vi "Pointcloud Paint.vi"(8 "error in (no error)":errorcluster, 11 "Pointcloud in":refnum<class "Pointcloud.lvclass">) -> (0 "error out":errorcluster, 2 "Pointcloud":refnum<vi>, 3 "Pointcloud out":refnum<class "Pointcloud.lvclass">)   [LabVIEW 2018, in "Pointcloud.lvclass"]
uses:
  Pointcloud.lvclass
  Pointcloud.lvclass/Pointcloud.ctl
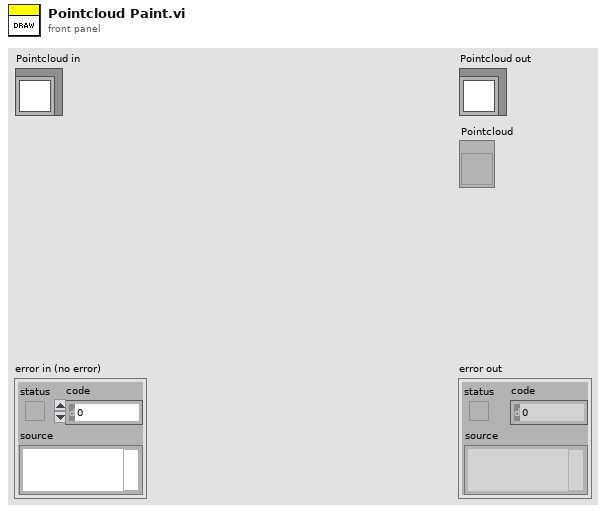
[diagram p1: front panel]
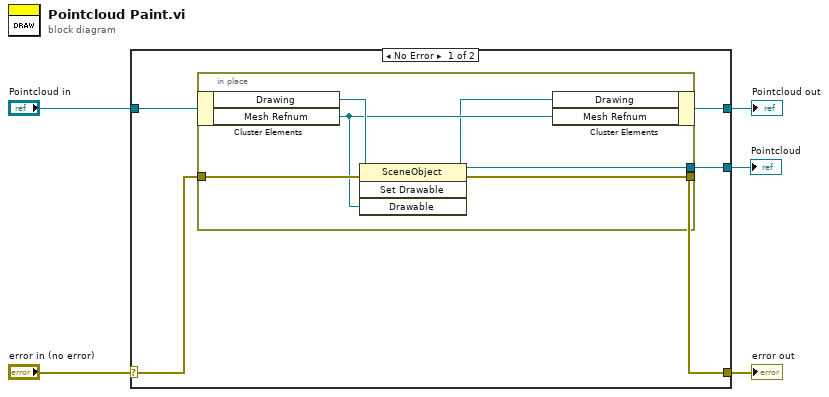
[diagram p0: block diagram]
diagram:
  n1 = case shown="No Error" "error in (no error)" {
    selector: "error in (no error)" -> [w8 w17]
    tunnel: [w7 w17] -> w4
    tunnel: [w9 w16] -> w2
    tunnel: "Pointcloud in" -> [w10 w16]
    tunnel: [w6 _] -> w1
    frame No Error {
      n2 = in-place {
        in-place-border: w8 -> [w14]
        in-place-border: [w12] -> w7
        in-place-border: [w11] -> w6
        n3 = in-place-cluster #1(w10) -> ("Drawing"=w15:refnum<vi>, "Mesh Refnum"=w13:refnum<vi>)
        n4 = invoke class="SceneObject" method="Set Drawable"(reference=w15, error in=w14, "Drawable"=w13) -> (reference out=w11:refnum<vi>, error out=w12:errorcluster)  [unwired: 1 in, 2 out]
        n5 = in-place-cluster #1("Drawing"=w11, "Mesh Refnum"=w13) -> (w9:refnum<class "Pointcloud.lvclass">)
      }
    }
    frame Error {
    }
  }
  "error out" <- w4
  "Pointcloud out" <- w2
  "Pointcloud" <- w1
